vi "fgv_stop_global.vi"(7 "cmd":T1) -> (3 "stop":bool)   [LabVIEW 2019]
uses:
  _ctrl/init-r-stop.ctl
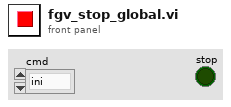
[diagram p1: front panel]
types:
  T1 = typedef "init-r-stop.ctl" = enum16{"ini", "read", "stop"}
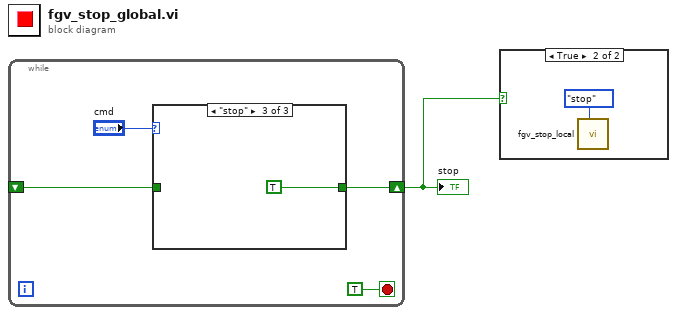
[diagram p0: block diagram]
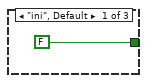
[diagram p3: hidden frame]
diagram:
  n1 = while {
    shift-right: [w3] -> w1
    shift-left: _ -> [w2]
    stop <- TRUE stop-if-true
    n2 = case shown="\"stop\"" "cmd" {
      tunnel: [FALSE w7 TRUE] -> w3
      tunnel: w2 -> [_ w7 _]
      frame "ini", Default {
      }
      frame "read" {
      }
      frame "stop" {
      }
    }
  }
  "stop" <- w1
  n3 = case shown="True" w1 {
    frame False {
    }
    frame True {
      n4 = call "fgv_stop_local.vi"("cmd"=init-r-stop."stop") -> ()  [unwired: 9 in, 2 out]
    }
  }
